vi "find_contours.vi"(11 "image in":T1) -> (2 "Source Image Points":cluster{"X":dbl, "Y":dbl}[](array[cluster]), 3 "image out":T1)   [LabVIEW 2017]
uses:
  <vilib>/vision/Image Controls.llb/IMAQ Image.ctl
  <vilib>/vision/Contour.llb/IMAQ Contour Curve Extraction.ctl
  <vilib>/vision/Contour.llb/IMAQ Connect Range Setting.ctl
  <vilib>/vision/NI_Vision_Development_Module.lvlib
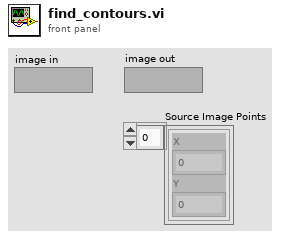
[diagram p1: front panel]
types:
  T1 = typedef "IMAQ Image.ctl" = refnum<image>
  T2 = enum16{"Rect Left To Right", "Rect Right To Left", "Rect Top To Bottom", "Rect Bottom To Top", "Annulus Inner To Outer", "Annulus Outer To Inner", "Annulus Start Angle To End Angle", "Annulus End Angle To Start Angle"}
  T3 = typedef "IMAQ Connect Range Setting.ctl" = cluster{"Match Constraints":u32, "Min":dbl, "Max":dbl}
  T4 = cluster{"Global Rectangle":i32[], "Contours":cluster{"ID":enum32{"External", "Internal"}, "Type":u32, "Coordinates":i32[]}[]}
  T5 = typedef "IMAQ Contour Curve Extraction.ctl" = cluster{"Extraction Mode":u32, "Edge Threshold":i32, "Edge Filter Size":u32, "Min Length":i32, "Search Step Size":i32, "Max Endpoint Gap":i32, "Subpixel":bool}
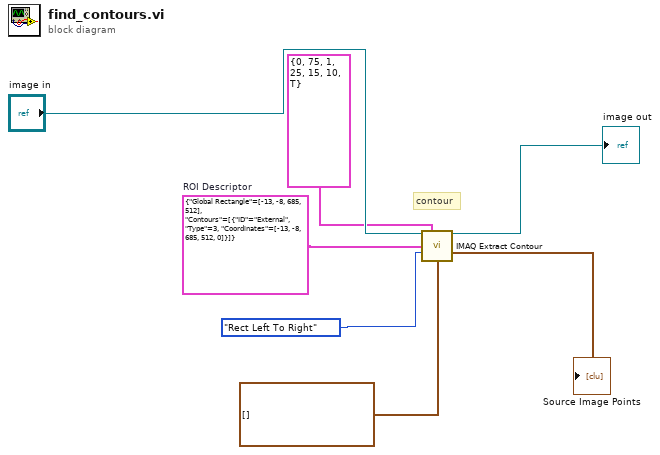
[diagram p0: block diagram]
diagram:
  w4 = T4 {"Global Rectangle"=[-13, -8, 685, 512], "Contours"=[{"ID"=enum."External", "Type"=3, "Coordinates"=[-13, -8, 685, 512, 0]}]}  # ROI Descriptor
  # "contour"
  n1 = call "IMAQ Extract Contour"("Source Image"="image in", "Curve Extraction"=T5 {"Extraction Mode"=0, "Edge Threshold"=75, "Edge Filter Size"=1, "Min Length"=25, "Search Step Size"=15, "Max Endpoint Gap"=10, "Subpixel"=TRUE}, "ROI Descriptor"=w4, "Search Direction"=T2."Rect Left To Right", "Curve Connection"=T3[] []) -> ("Source Image Out"=→"image out":T1, "Source Image Points"=→"Source Image Points":cluster{"X":dbl, "Y":dbl}[])  [unwired: 3 in, 6 out]
